vi "Gamepad.vi"() -> (2 "Stop":bool, 3 "Switch":bool)   [LabVIEW 2015]
uses:
  <vilib>/Utility/inputDevices.llb/joystickAcquire.vi
  <vilib>/Utility/inputDevices.llb/closeJoystick.vi
panel:
  in  "switch":bool
  out "Logitech Gamepad":T1 {"Axis 1" scale=-1.0..1.0; "Axis 2" scale=-1.0..1.0; "Axis 3" scale=-1.0..1.0; "Axis 4" scale=-1.0..1.0; "POV 1" scale=0.0..360.0}
  in  "stop":bool
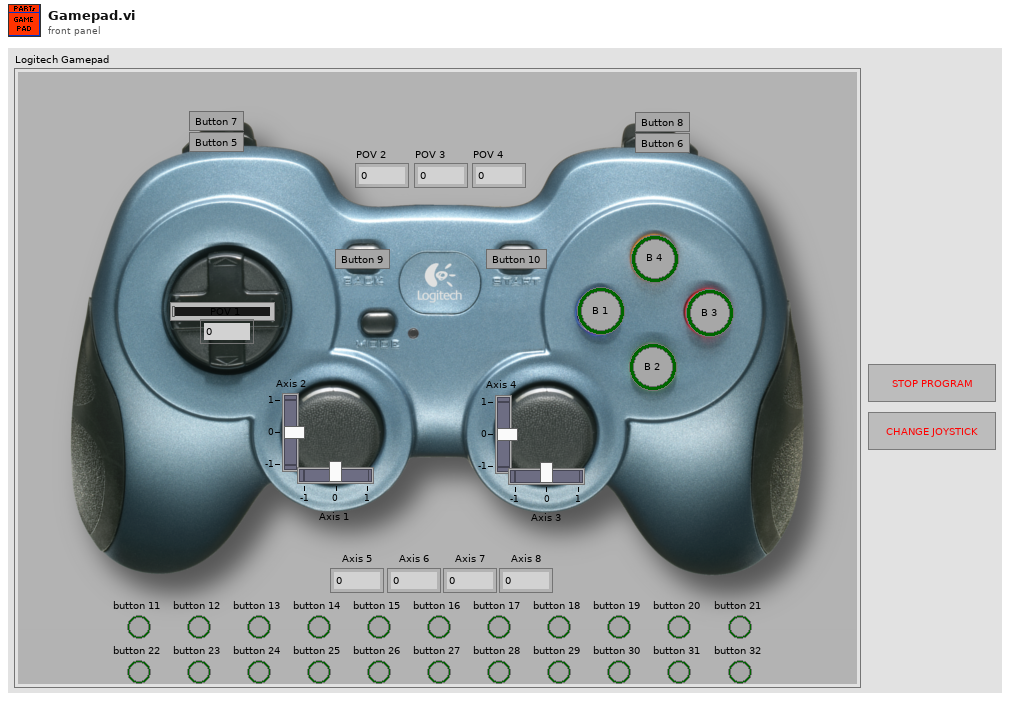
[diagram p1: front panel]
types:
  T1 = cluster{"Axis 1":i32, "Axis 2":i32, "Axis 3":i32, "Axis 4":i32, "Axis 5":i32, "Axis 6":i32, "Axis 7":i32, "Axis 8":i32, "B 1":bool, "B 2":bool, "B 3":bool, "B 4":bool, "button 5":bool, "button 6":bool, "button 7":bool, "button 8":bool, "button 9":bool, "button 10":bool, "button 11":bool, "button 12":bool, "button 13":bool, "button 14":bool, "button 15":bool, "button 16":bool, "button 17":bool, "button 18":bool, "button 19":bool, "button 20":bool, "button 21":bool, "button 22":bool, "button 23":bool, "button 24":bool, "button 25":bool, "button 26":bool, "button 27":bool, "button 28":bool, "button 29":bool, "button 30":bool, "button 31":bool, "button 32":bool, "POV 1":i32, "POV 2":i32, "POV 3":i32, "POV 4":i32}
  T2 = cluster{"X axis":i32, "Y axis":i32, "Z axis":i32, "X axis rotation":i32, "Y axis rotation":i32, "Z axis rotation":i32, "U axis":i32, "V axis":i32}
  T3 = cluster{"button 1":bool, "button 2":bool, "button 3":bool, "button 4":bool, "button 5":bool, "button 6":bool, "button 7":bool, "button 8":bool, "button 9":bool, "button 10":bool, "button 11":bool, "button 12":bool, "button 13":bool, "button 14":bool, "button 15":bool, "button 16":bool, "button 17":bool, "button 18":bool, "button 19":bool, "button 20":bool, "button 21":bool, "button 22":bool, "button 23":bool, "button 24":bool, "button 25":bool, "button 26":bool, "button 27":bool, "button 28":bool, "button 29":bool, "button 30":bool, "button 31":bool, "button 32":bool}
  T4 = cluster{"pov 1":i32, "pov 2":i32, "pov 3":i32, "pov 4":i32}
  T5 = cluster{"X axis":i32, "Y axis":i32, "Z axis":i32, "X axis rotation":i32, "Y axis rotation":i32, "Z axis rotation":i32, "U axis":i32, "V axis":i32, "button 1":bool, "button 2":bool, "button 3":bool, "button 4":bool, "button 5":bool, "button 6":bool, "button 7":bool, "button 8":bool, "button 9":bool, "button 10":bool, "button 11":bool, "button 12":bool, "button 13":bool, "button 14":bool, "button 15":bool, "button 16":bool, "button 17":bool, "button 18":bool, "button 19":bool, "button 20":bool, "button 21":bool, "button 22":bool, "button 23":bool, "button 24":bool, "button 25":bool, "button 26":bool, "button 27":bool, "button 28":bool, "button 29":bool, "button 30":bool, "button 31":bool, "button 32":bool, "pov 1":i32, "pov 2":i32, "pov 3":i32, "pov 4":i32}
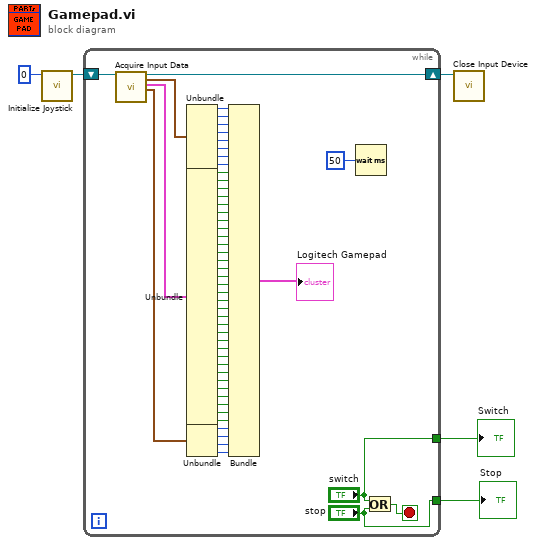
[diagram p0: block diagram]
diagram:
  n1 = call <vilib>:"Initialize Joystick.vi"("device index"=0) -> ("device ID"=w5:refnum<k1>)  [unwired: 9 in, 1 out]
  n2 = while {
    shift-right: [w58] -> w4
    shift-left: w5 -> [w59]
    tunnel: ["stop"] -> w3
    tunnel: ["switch"] -> w2
    stop <- w57 stop-if-true
    n3 = call-poly <vilib>:"Acquire Input Data.vi"("device ID"=w59) -> ("device ID"=w58:refnum<k1>, "axis info"=w54:T2, "button info"=w53:T3, "direction info"=w52:T4)  [unwired: 14 in, 1 out]
    n4 = Unbundle(w54) -> ("X axis"=w51:i32, "Y axis"=w50:i32, "Z axis"=w49:i32, "X axis rotation"=w48:i32, "Y axis rotation"=w47:i32, "Z axis rotation"=w46:i32, "U axis"=w45:i32, "V axis"=w44:i32)
    n5 = Unbundle(w53) -> ("button 1"=w43:bool, "button 2"=w42:bool, "button 3"=w41:bool, "button 4"=w40:bool, "button 5"=w39:bool, "button 6"=w38:bool, "button 7"=w37:bool, "button 8"=w36:bool, "button 9"=w35:bool, "button 10"=w34:bool, "button 11"=w33:bool, "button 12"=w32:bool, "button 13"=w31:bool, "button 14"=w30:bool, "button 15"=w29:bool, "button 16"=w28:bool, "button 17"=w27:bool, "button 18"=w26:bool, "button 19"=w25:bool, "button 20"=w24:bool, "button 21"=w23:bool, "button 22"=w22:bool, "button 23"=w21:bool, "button 24"=w20:bool, "button 25"=w19:bool, "button 26"=w18:bool, "button 27"=w17:bool, "button 28"=w16:bool, "button 29"=w15:bool, "button 30"=w14:bool, "button 31"=w13:bool, "button 32"=w12:bool)
    n6 = Unbundle(w52) -> ("pov 1"=w11:i32, "pov 2"=w10:i32, "pov 3"=w9:i32, "pov 4"=w8:i32)
    n7 = Bundle("X axis"=w51, "Y axis"=w50, "Z axis"=w49, "X axis rotation"=w48, "Y axis rotation"=w47, "Z axis rotation"=w46, "U axis"=w45, "V axis"=w44, "button 1"=w43, "button 2"=w42, "button 3"=w41, "button 4"=w40, "button 5"=w39, "button 6"=w38, "button 7"=w37, "button 8"=w36, "button 9"=w35, "button 10"=w34, "button 11"=w33, "button 12"=w32, "button 13"=w31, "button 14"=w30, "button 15"=w29, "button 16"=w28, "button 17"=w27, "button 18"=w26, "button 19"=w25, "button 20"=w24, "button 21"=w23, "button 22"=w22, "button 23"=w21, "button 24"=w20, "button 25"=w19, "button 26"=w18, "button 27"=w17, "button 28"=w16, "button 29"=w15, "button 30"=w14, "button 31"=w13, "button 32"=w12, "pov 1"=w11, "pov 2"=w10, "pov 3"=w9, "pov 4"=w8) -> (→"Logitech Gamepad":T5)  [unwired: 1 in]
    n8 = Wait (ms)(milliseconds to wait=u32 50) -> ()  [unwired: 1 out]
    n9 = Or(x="switch", y="stop") -> (x .or. y?=w57:bool)
  }
  "Stop" <- w3
  "Switch" <- w2
  n10 = call-poly <vilib>:"Close Input Device.vi"("device ID"=w4) -> ()  [unwired: 9 in, 1 out]
